vi "Set DAC Offset.vi"(4 "error in (no error)":errorcluster, 5 "DAC Offset (0)":dbl min=-10.0 max=10.0 format="%.6g", 6 "Axis (1)":i32=1 min=1 max=3, 7 "VISA resource name":refnum<visa-resource-name>) -> (0 "error out":errorcluster, 3 "VISA resource name out":refnum<visa-resource-name>)   [LabVIEW 2010, in "Newport ESP301.lvlib"]
doc: "This command is used to set the DAC offset compensation for the specified DAC channel. There are two DAC channels associated with every axis: DAC channels 1 and 2 are associated with axis #1, DAC channels 3 and 4 with axis #2 etc.\nIn order for the DAC offset to take affect, this command must be followed by the ASCII command, UF (Update Filter). This offset may be saved to non-volatile flash memory by issuing the ASCII command, SM. This will cause the DSP to automatically use the saved value after system reset or reboot.\n<B>Note:</B> DAC offset compensation is necessary on servo axes to prevent motor drift during motor off conditions."
uses:
  <userlib>/Newport ESP301/Newport ESP301.lvlib
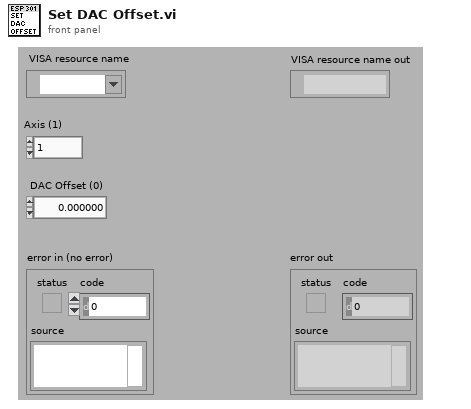
[diagram p1: front panel]
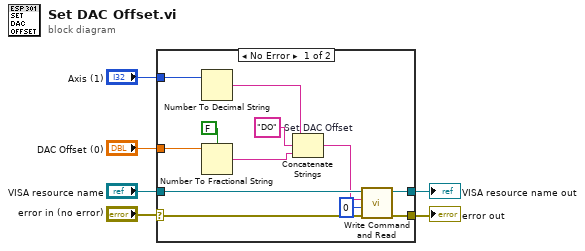
[diagram p0: block diagram]
diagram:
  n1 = case shown="No Error" "error in (no error)" {
    selector: "error in (no error)" -> [w15 w20]
    tunnel: [w17 w20] -> w6
    tunnel: "VISA resource name" -> [w18 w19]
    tunnel: [w16 w19] -> w5
    tunnel: "DAC Offset (0)" -> [w14 _]
    tunnel: "Axis (1)" -> [w13 _]
    frame No Error {
      w12 = "DO"  # Set DAC Offset
      n2 = Number To Decimal String(number=w13) -> (decimal integer string=w11:string)  [unwired: 1 in]
      n3 = Number To Fractional String(use system decimal point (T)=FALSE ("utiliser le séparateur décimal du système (V)"), number=w14) -> (F-format string=w10:string)  [unwired: 2 in]
      n4 = Concatenate Strings(w11, w12, w10) -> (w9:string)
      n5 = call <userlib>:"Write Command and Read.vi"("error in (no error)"=w15, "Bytes to read (100)"=u32 0, "Command"=w9, "VISA resource name"=w18) -> ("error out"=w17:errorcluster, "VISA resource name out"=w16:refnum<visa-resource-name>)  [unwired: 3 in, 1 out]
    }
    frame Error {
    }
  }
  "error out" <- w6
  "VISA resource name out" <- w5
